vi "set_output_voltage.vi"(8 "error in (no error)":errorcluster, 10 "output value":dbl[unit], 11 "DAQmxAnalogOut in":refnum<class "AnalogOutDL101207DAQmx.lvclass">) -> (0 "error out":errorcluster, 3 "DAQmxAnalogOut out":refnum<class "AnalogOutDL101207DAQmx.lvclass">)   [LabVIEW 2010, in "AnalogOutDL101207DAQmx.lvclass"]
uses:
  AnalogOutDL101207DAQmx.lvclass
  AnalogOutDL101207DAQmx.lvclass/AnalogOutDL101207DAQmx.ctl
  <vilib>/DAQmx/write.llb/DAQmx Write (Analog DBL 1Chan 1Samp).vi
  <vilib>/daqmx/miscellaneous.llb/DAQmx Fill In Error Info.vi
  common/classes/ErrorController/ErrorController/class_data.vi
  common/classes/ErrorController/ErrorController/ErrorController.lvclass
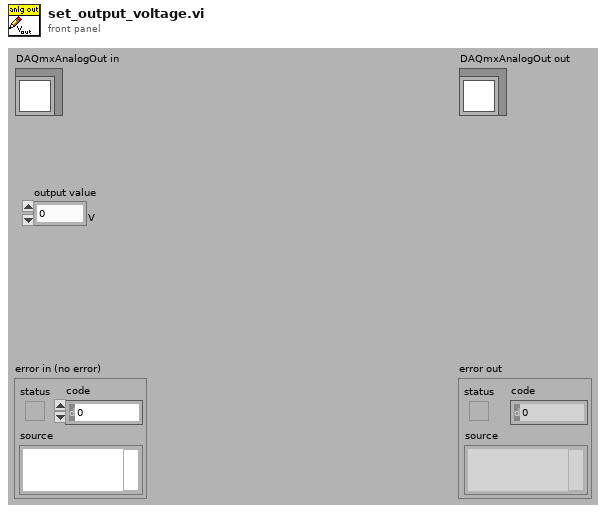
[diagram p1: front panel]
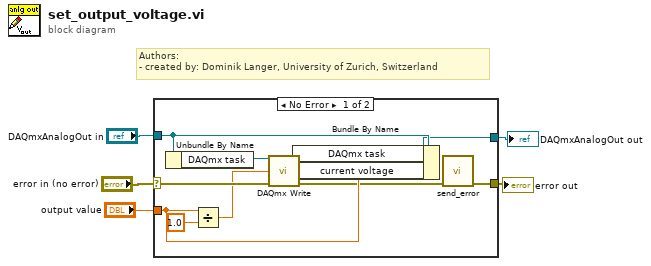
[diagram p0: block diagram]
diagram:
  # "Authors: \n- created by: Dominik Langer, University of Zurich, Switzerland"
  n1 = case shown="No Error" "error in (no error)" {
    selector: "error in (no error)" -> [w14 w17]
    tunnel: [w6 w17] -> w4
    tunnel: [w11 w16] -> w2
    tunnel: "DAQmxAnalogOut in" -> [w12 w16]
    tunnel: "output value" -> [w8 _]
    frame No Error {
      n2 = Unbundle By Name(w12) -> ("DAQmx task"=w15:refnum<k21>)
      n3 = Divide(x=w8, y=dbl[unit] 1.0) -> (x/y=w9:dbl)
      n4 = call-poly <vilib>:"DAQmx Write.vi"("task/channels in"=w15, "data"=w9, "error in"=w14) -> ("task out"=w13:refnum<k21>, "error out"=w7:errorcluster)  [unwired: 1 in, 10 out]
      n5 = Bundle By Name(cluster=w12, "DAQmx task"=w13, "current voltage"=w8) -> (w11:refnum<class "AnalogOutDL101207DAQmx.lvclass">)
      n6 = call "send_error.vi"("error in (no error)"=w7) -> ("error out"=w6:errorcluster)  [unwired: 10 in]
    }
    frame Error {
    }
  }
  "error out" <- w4
  "DAQmxAnalogOut out" <- w2
